vi "DSF.Engine.Transceiver Thread.Send Base Pointer.vi"(8 "error in (no error)":errorcluster, 9 "engine size":u64, 10 "engine base address":u64 format="%.0x", 11 "Transceiver Interface in":refnum<class "DSF.Engine.Interface.Transceiver.lvclass">) -> (0 "error out":errorcluster, 3 "Transceiver Interface out":refnum<class "DSF.Engine.Interface.Transceiver.lvclass">)   [LabVIEW 2017, in "DSF.Engine.lvlib" / "DSF.Engine.Transceiver Thread.lvclass"]
uses:
  DSF.Engine.Transceiver Thread.lvclass
  Interface/DSF.Engine.Interface.Transceiver.lvclass
  Interface/DSF.Engine.Interface.Transceiver.Command Data.ctl
  Interface/DSF.Engine.Interface.Transceiver.Command.ctl
  Interface/DSF.Engine.Interface.Transceiver.Command Parameters.ctl
  Interface/DSF.Engine.Interface.Transceiver.Response.ctl
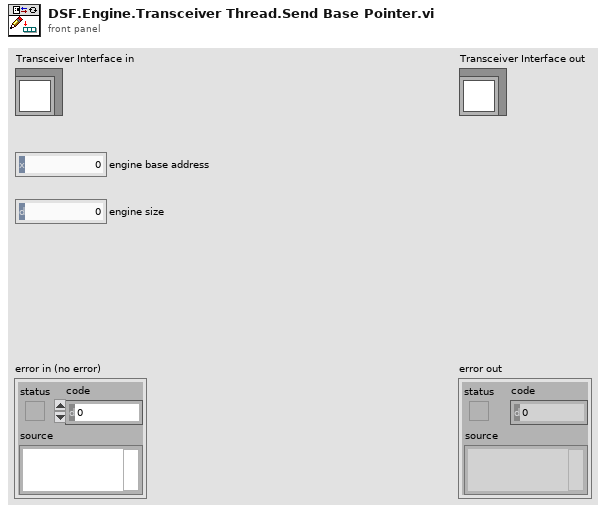
[diagram p1: front panel]
types:
  T1 = typedef "DSF.Engine.lvlib/DSF.Engine.Interface.Transceiver.lvclass/DSF.Engine.Interface.Transceiver.Command Data.ctl" = cluster{"Command":T2, "Command Parameters":T3}
  T2 = typedef "DSF.Engine.lvlib/DSF.Engine.Interface.Transceiver.lvclass/DSF.Engine.Interface.Transceiver.Command.ctl" = enum8{"Set Base Pointer", "Rx", "Tx", "Shutdown"}
  T3 = typedef "DSF.Engine.lvlib/DSF.Engine.Interface.Transceiver.lvclass/DSF.Engine.Interface.Transceiver.Command Parameters.ctl" = cluster{"arg1":u64, "arg2":u64}
  T4 = typedef "DSF.Engine.lvlib/DSF.Engine.Interface.Transceiver.lvclass/DSF.Engine.Interface.Transceiver.Response.ctl" = enum8{"General Ack", "Shutting Down"}
  T5 = typedef "DSF.Engine.lvlib/DSF.Engine.Interface.Transceiver.lvclass/DSF.Engine.Interface.Transceiver.Response Data.ctl" = cluster{"Response":T4, "Response Parameters":T6}
  T6 = typedef "DSF.Engine.lvlib/DSF.Engine.Interface.Transceiver.lvclass/DSF.Engine.Interface.Transceiver.Response Parameters.ctl" = cluster{"arg1":u64, "arg2":u64}
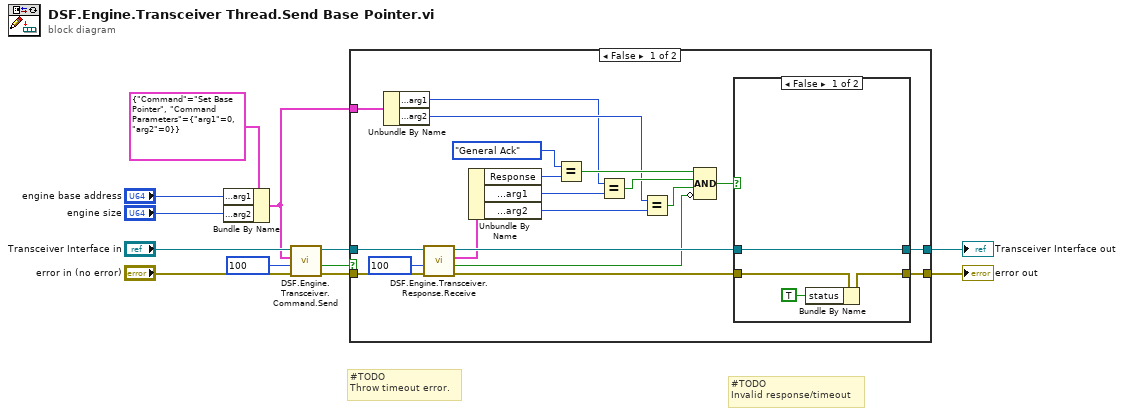
[diagram p0: block diagram]
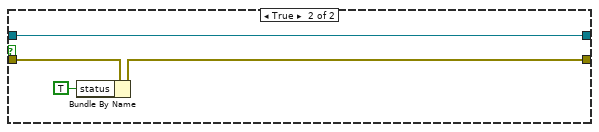
[diagram p3: hidden frame]
diagram:
  # "#TODO\nInvalid response/timeout"
  # "#TODO\nThrow timeout error."
  n1 = Bundle By Name(cluster=T1 {"Command"=enum."Set Base Pointer", "Command Parameters"={"arg1"=0, "arg2"=0}} ("command"), "Command Parameters.arg1"="engine base address", "Command Parameters.arg2"="engine size") -> (w1:T1)
  n2 = call "DSF.Engine.Transceiver.Command.Send.vi"("error in (no error)"="error in (no error)", "timeout in ms (0)"=100, "command"=w1, "Transceiver Interface in"="Transceiver Interface in") -> ("error out"=w10:errorcluster, "timed out?"=w11:bool, "Transceiver Interface out"=w9:refnum<class "DSF.Engine.Interface.Transceiver.lvclass">)  [unwired: 5 in]
  n3 = case shown="False" w11 {
    tunnel: w10 -> [w31 w42]
    tunnel: w9 -> [w32 w39]
    tunnel: [w24 w40] -> w6
    tunnel: [w22 w39] -> w5
    tunnel: w1 -> [w19 _]
    frame False {
      n4 = Unbundle By Name(w19) -> ("Command Parameters.arg1"=w13:u64, "Command Parameters.arg2"=w14:u64)
      n5 = call "DSF.Engine.Transceiver.Response.Receive.vi"("error in (no error)"=w31, "timeout in ms (0)"=100, "Transceiver Thread in"=w32) -> ("error out"=w25:errorcluster, "timed out?"=w20:bool, "response"=w21:T5, "Transceiver Thread out"=w23:refnum<class "DSF.Engine.Interface.Transceiver.lvclass">)  [unwired: 5 in]
      n6 = Unbundle By Name(w21) -> ("Response"=w29:T4, "Response Parameters.arg1"=w18:u64, "Response Parameters.arg2"=w17:u64)
      n7 = Equal?(x=DSF.Engine.Interface.Transceiver.Response."General Ack", y=w29) -> (x = y?=w27:bool)
      n8 = Equal?(x=w13, y=w18) -> (x = y?=w16:bool)
      n9 = Equal?(x=w14, y=w17) -> (x = y?=w15:bool)
      n10 = Compound Arithmetic op=AND(w27, w16, w15, invert w20) -> (w26:bool)
      n11 = case shown="False" w26 {
        tunnel: w25 -> [w36 w38]
        tunnel: [w34 w38] -> w24
        tunnel: w23 -> [w33 w37]
        tunnel: [w33 w37] -> w22
        frame False {
          n12 = Bundle By Name(cluster=w36, "status"=TRUE) -> (w34:errorcluster)
        }
        frame True {
        }
      }
    }
    frame True {
      n13 = Bundle By Name(cluster=w42, "status"=TRUE) -> (w40:errorcluster)
    }
  }
  "error out" <- w6
  "Transceiver Interface out" <- w5
